vi "main.vi"() -> ()   [LabVIEW 2025]
uses:
  <userlib>/_NEVSTOP/Communicable State Machine(CSM)/Communicable State Machine.lvlib
  9e748aeb-3768-48be-8dba-7a0c5cfaea59.vi
  93a68443-ce49-4d48-b9a9-034adad3285b.vi
  780328b8-20a8-4e4e-91e5-c479b507fea7.vi
  <userlib>/_NEVSTOP/Communicable State Machine(CSM)/_Polymophic/Build Status Broadcast Message.vi
panel:
  out "Monitor":picture
  out "Error Occurred":errorcluster
  out "State History":string
  in  "Name (\"\" to Use UUID)":string="main"
  in  "Exit":bool
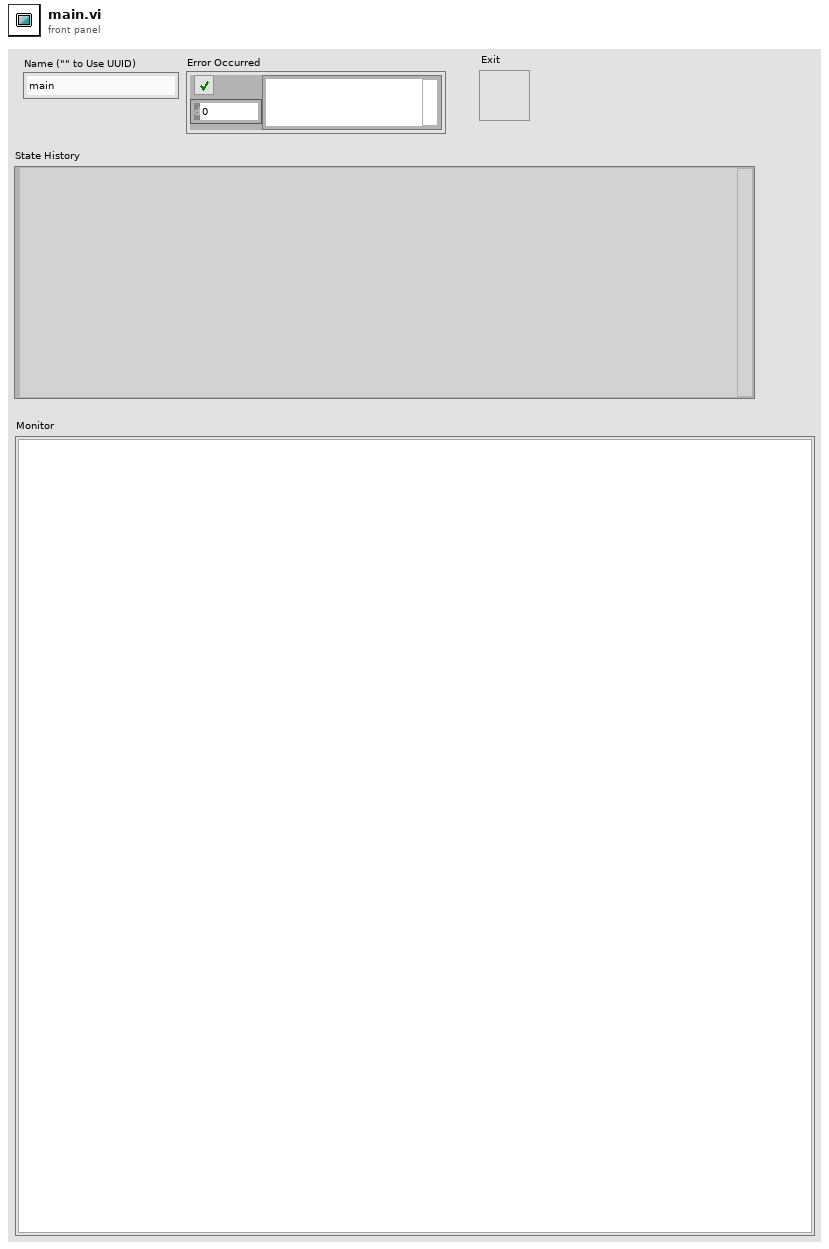
[diagram p1: front panel]
types:
  T1 = enum32{"Invalid", "Standard", "Closed", "Hidden", "Minimized", "Maximized"}
  T2 = enum32{"invalid app kind", "Development System", "Run Time System", "Student Edition", "Embedded LabVIEW", "Evaluation", "Custom"}
  T3 = cluster{"left":i16, "top":i16, "right":i16, "bottom":i16}
  T4 = typedef "Communicable State Machine.lvlib/_CSM_Response Source Message.ctl" = cluster{"‘State":string, "’Arguments":string, "’Error":errorcluster}
  T5 = typedef "eventvkey.ctl" = enum16{"ASCII", "Enter", "Return", "Shift", "Ctrl", "Alt", "Cmd", "Opt", "Caps", "NumLock", "Clear", "Break", "Up", "Down", "Left", "Right", "Insert", "Delete", "Home", "End", "PageUp", "PageDown", "Escape", "Help", "Pause", "ScrollLock", "F1", "F2", "F3", "F4", "F5", "F6", "F7", "F8", "F9", "F10", "F11", "F12", "F13", "F14", "F15", "F16", "F17", "F18", "F19", "F20", "F21", "F22", "F23", "F24", "Play", "VolumeUp", "VolumeDown", "Mute", "Two Byte Char"}
  T6 = cluster{"Current VI Reference":refnum<vi>, "Close Panel on Exit?":bool}
  T7 = cluster{"Core":cluster{"Current VI Reference":refnum<vi>, "Close Panel on Exit?":bool}, "player":cluster{"left":i16, "top":i16, "right":i16, "bottom":i16}, "Top Left Walll":cluster{"x":i16, "y":i16}[], "Top Right Walll":cluster{"x":i16, "y":i16}[], "Down Left Walll":cluster{"x":i16, "y":i16}[], "Down RightWalll":cluster{"x":i16, "y":i16}[], "Monitor":picture, "Gate Up":cluster{"left":i16, "top":i16, "right":i16, "bottom":i16}, "Gate Down":cluster{"left":i16, "top":i16, "right":i16, "bottom":i16}, "Gate Left":cluster{"left":i16, "top":i16, "right":i16, "bottom":i16}, "Gate Right":cluster{"left":i16, "top":i16, "right":i16, "bottom":i16}, "Gate Condition":bool[], "Level":i32}
  T8 = cluster{"left":i16, "top":i16, "right":i16, "bottom":i16}[]
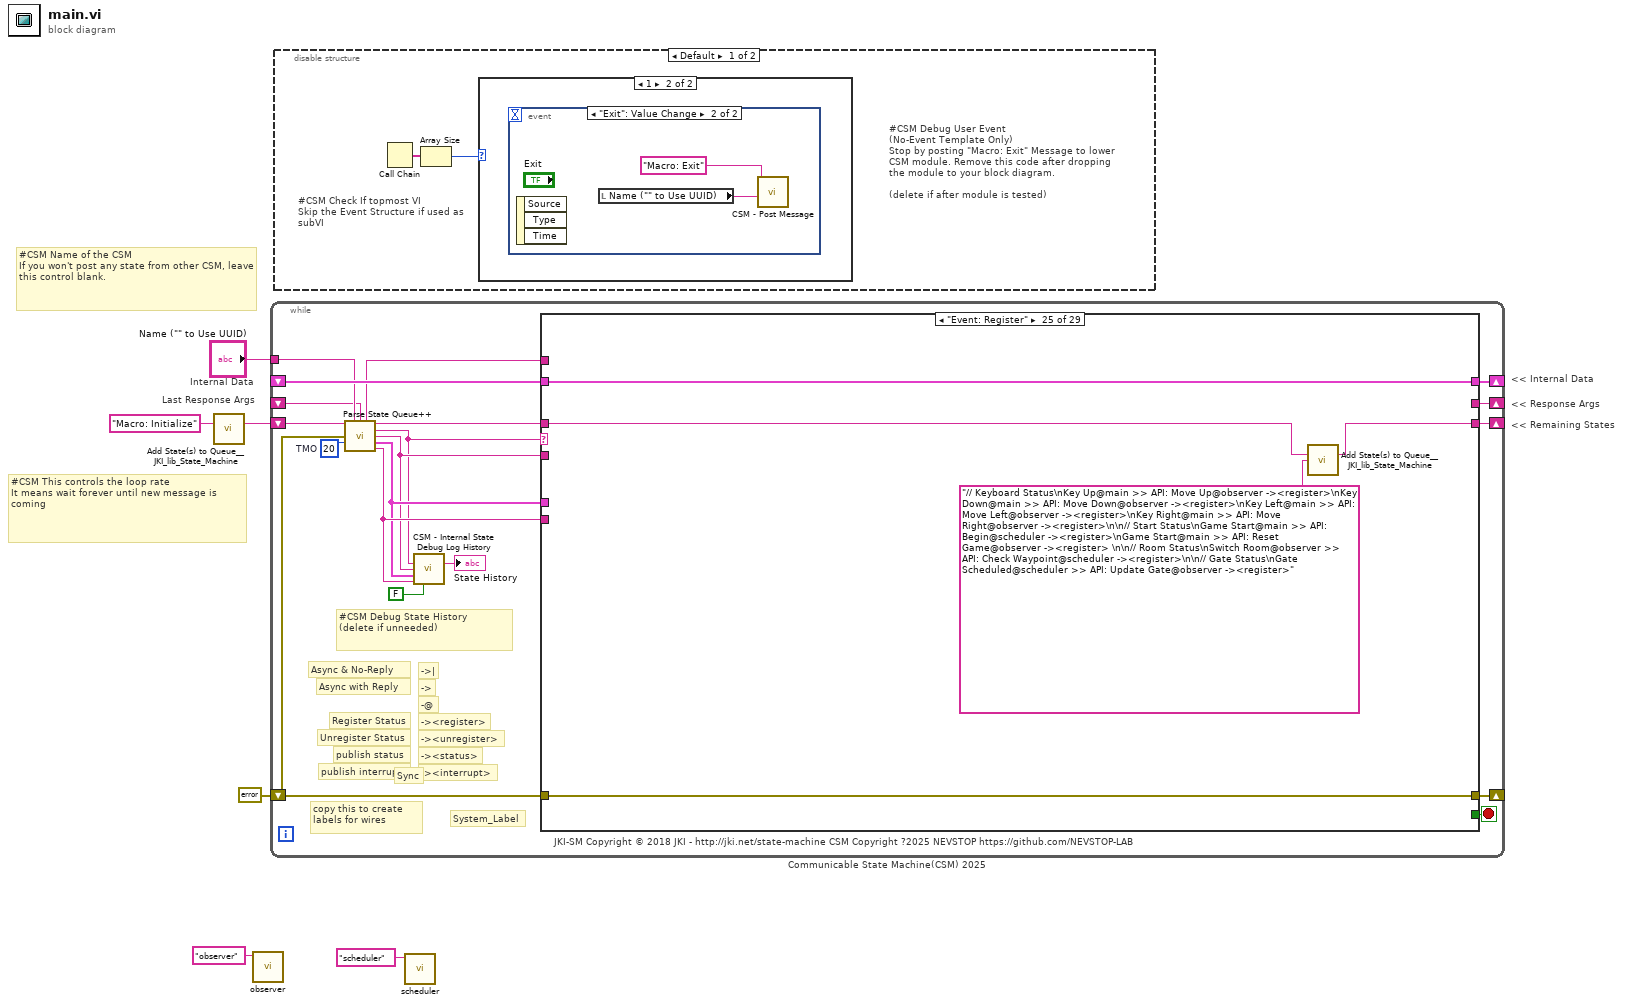
[diagram p0: block diagram]
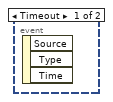
[diagram p3: hidden frame]
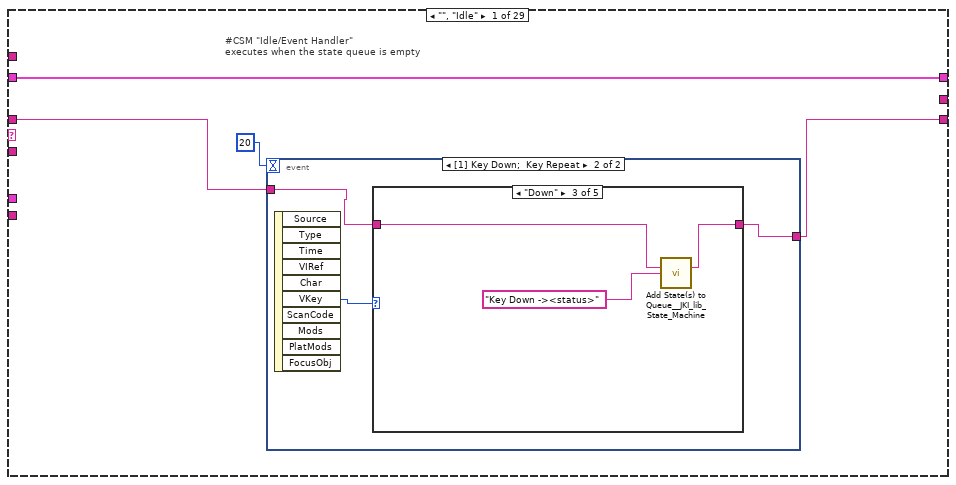
[diagram p5: hidden frame]
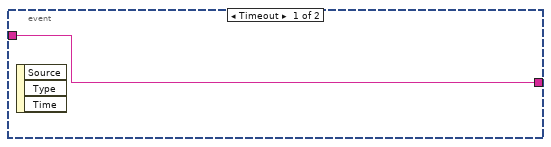
[diagram p6: hidden frame]
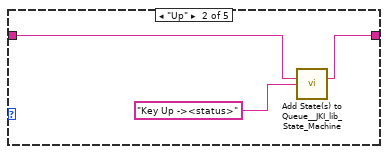
[diagram p8: hidden frame]
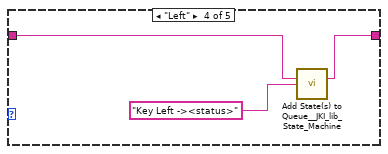
[diagram p9: hidden frame]
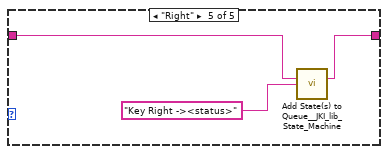
[diagram p10: hidden frame]
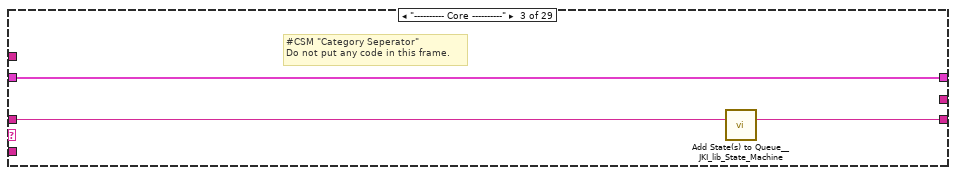
[diagram p12: hidden frame]
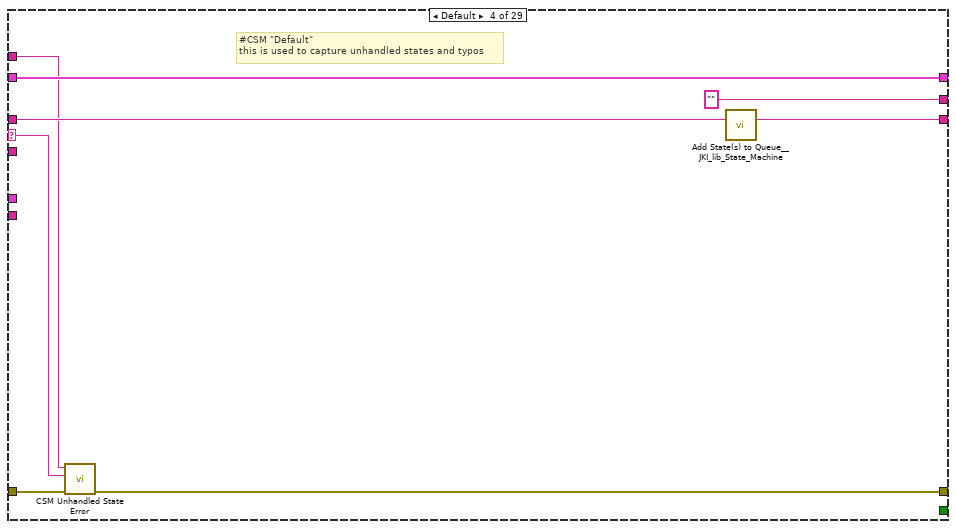
[diagram p13: hidden frame]
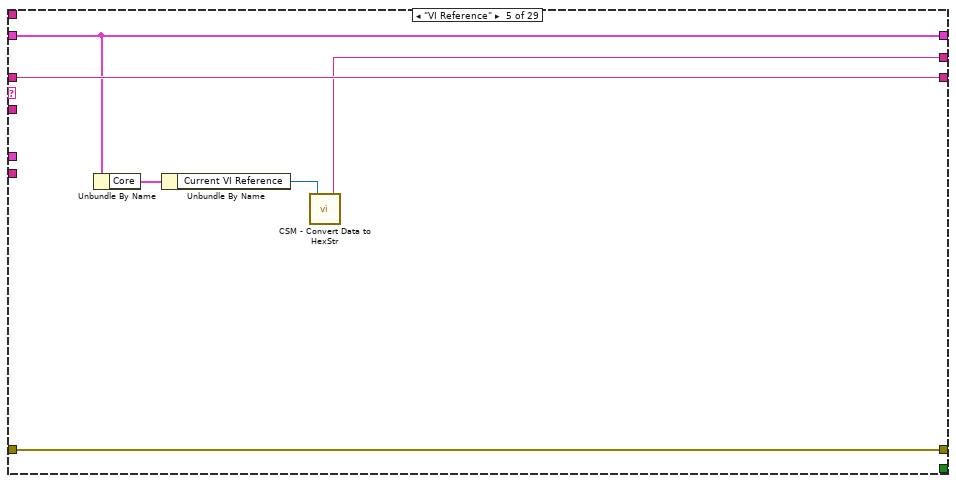
[diagram p14: hidden frame]
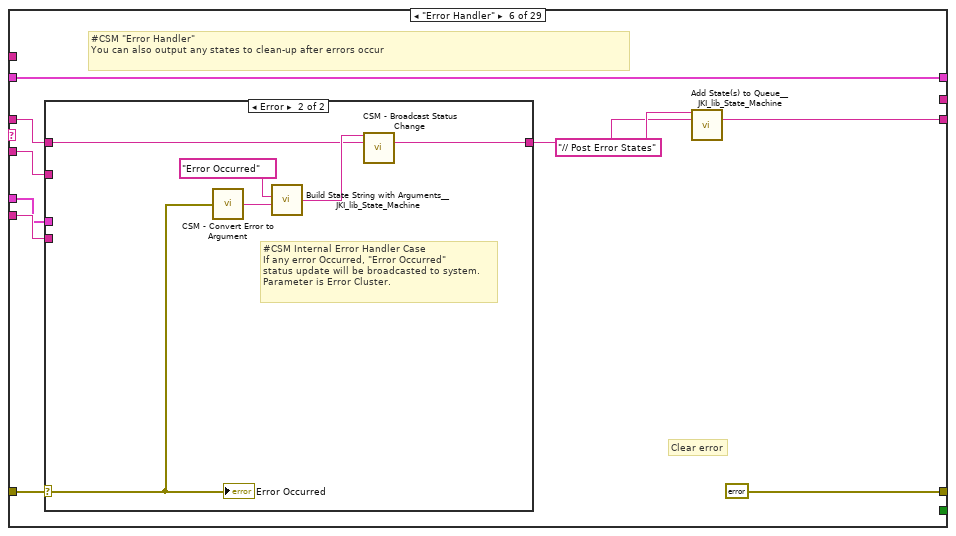
[diagram p15: hidden frame]
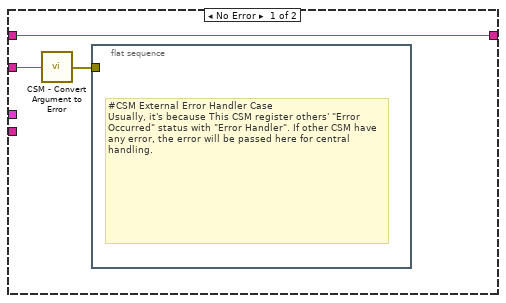
[diagram p16: hidden frame]
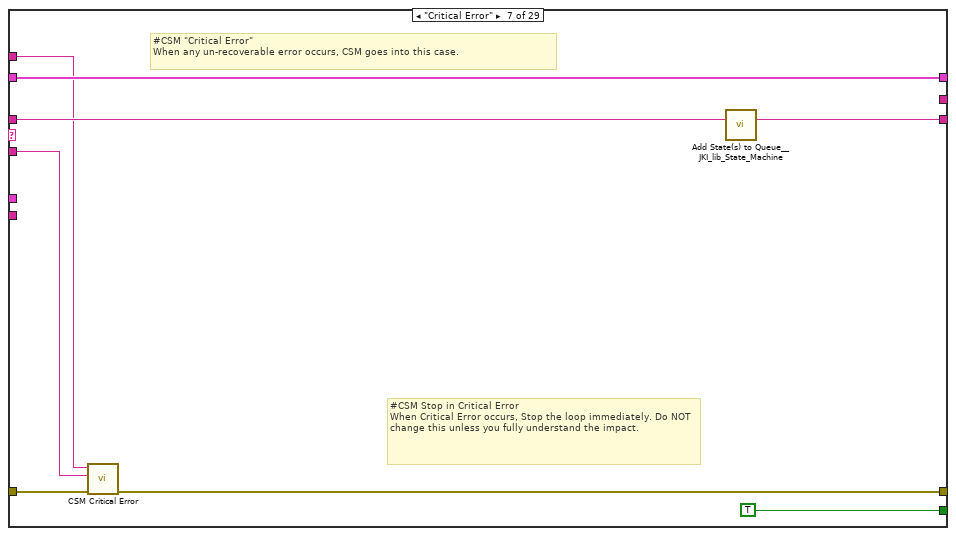
[diagram p17: hidden frame]
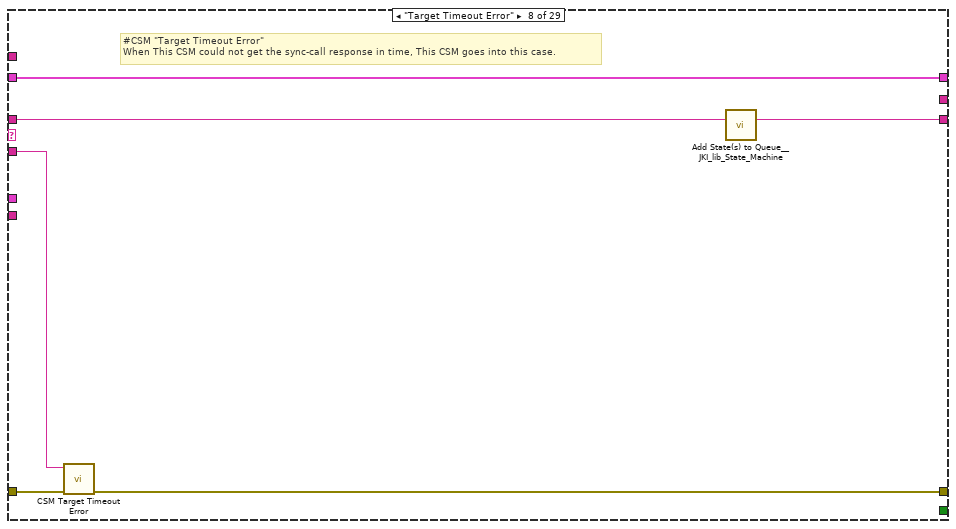
[diagram p18: hidden frame]
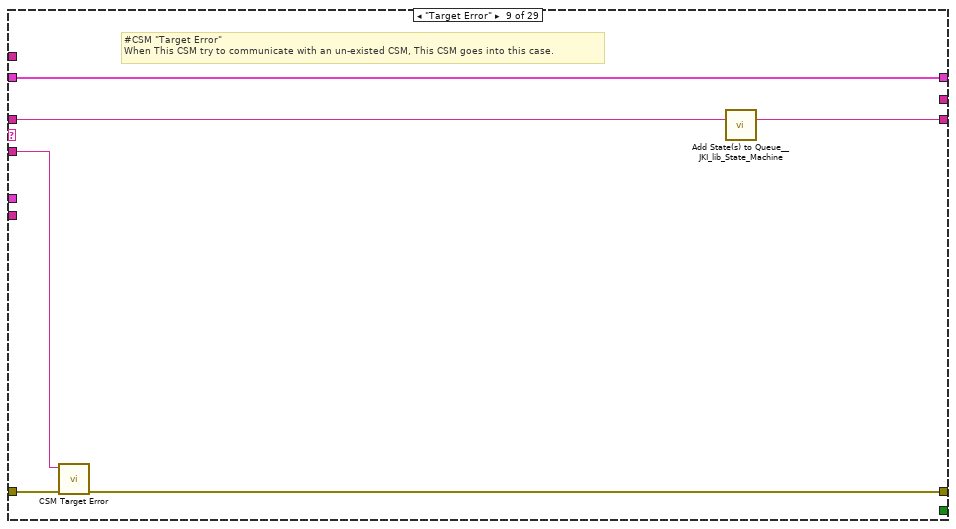
[diagram p19: hidden frame]
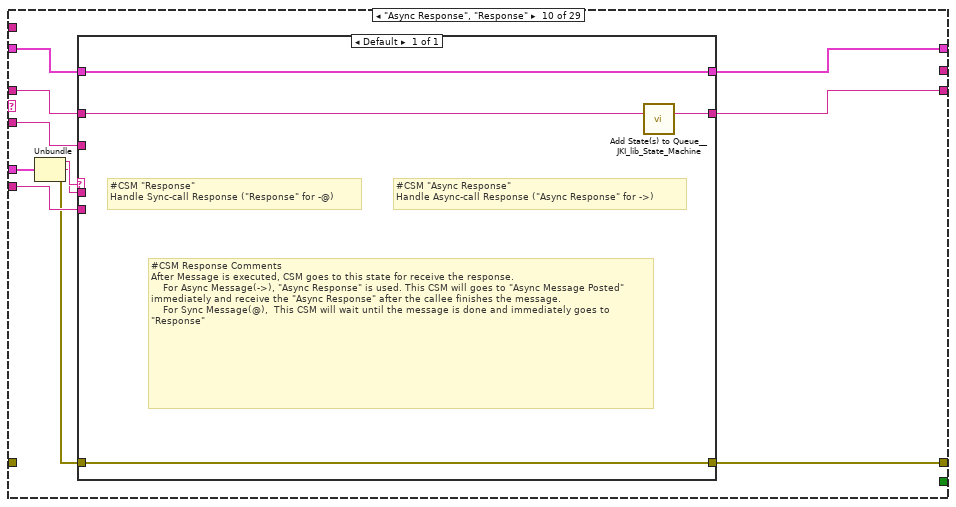
[diagram p20: hidden frame]
diagram:
  # "Last Response Args"
  # "Internal Data"
  # "#CSM Name of the CSM\nIf you won't post any state from other CSM, leave this control blank."
  # "#CSM This controls the loop rate\nIt means wait forever until new message is coming"
  # "<< Internal Data"
  # "<< Response Args"
  # "<< Remaining States"
  n1 = call <vilib>:"Add State(s) to Queue__JKI_lib_State_Machine.vi"("State(s) in (\"\")"="Macro: Initialize" ("Init State(\"Macro: Initialize\")")) -> ("States Out"=w3:string)  [unwired: 14 in]
  n2 = call "observer.vi"("Name (\"\" to Use UUID)"="observer" ("Name (\"\" to Use UUID)")) -> ()  [unwired: 11 in]
  n3 = while "Communicable State Machine(CSM) 2025" {
    shift-right: [w20] -> _
    shift-left: _ -> [w19]
    shift-right: [w23] -> _
    shift-left: errorcluster {"status"=FALSE, "code"=0, "source"=""} ("error out") -> [w9]
    shift-right: [w22] -> _
    shift-left: w3 -> [w24]
    tunnel: "Name (\"\" to Use UUID)" -> [w16]
    shift-right: [w17] -> _
    shift-left: _ -> [w11]
    stop <- w21 stop-if-true
    w18 = 20  # TMO
    # "#CSM Debug State History\n(delete if unneeded)"
    # "-><interrupt>"
    # "-><status>"
    # "-><unregister>"
    # "-><register>"
    # "-@"
    # "->"
    # "->|"
    # "publish interrupt"
    # "publish status"
    # "Unregister Status"
    # "Register Status"
    # "Sync"
    # "Async with Reply"
    # "Async & No-Reply"
    # "JKI-SM Copyright © 2018 JKI - http://jki.net/state-machine CSM Copyright ?2025 NEVSTOP https://github.com/NEVSTOP-LAB"
    # "copy this to create labels for wires"
    # "System_Label"
    n4 = call <userlib>:"Parse State Queue++.vi"("State Queue"=w24, "Name (\"\" to Use UUID)"=w16, "Response Arguments"=w11, "Previous Error"=w9, "Dequeue (1 ms)"=w18) -> ("Name Used"=w10:string, "Remaining States"=w25:string, "Current State"=w12:string, "Arguments"=w13:string, "Additional Information"=w14:T4, "Source CSM"=w15:string)  [unwired: 5 in]
    n5 = call <userlib>:"CSM - Internal State Debug Log History.vi"("State"=w12, "Arguments (\"\")"=w13, ">> Response Source Message >>"=w14, "Source (\"\")"=w15, "Enable Periodic State Filter? (T)"=FALSE) -> ("Debug Log"=→"State History":string)  [unwired: 10 in]
    n6 = case shown="\"Event: Register\"" w12 {
      selector: w12 -> [_ _ _ w55 _ _ _ _ _ _ _ _ _ _ _ _ _ _ _ _ _ _ _ _ _ _ _ _ _]
      tunnel: w25 -> [w27 w48 w51 w59 w64 w69 w92 w98 w104 w114 w121 w133 w137 w140 w156 w158 w164 w166 w168 w205 w209 w223 w230 w232 w236 w240 w243 w252 w261]
      tunnel: w13 -> [_ _ _ _ _ w68 w88 w95 w101 w108 _ _ _ _ _ _ _ _ _ _ _ _ _ _ _ _ _ w250 w259]
      tunnel: w19 -> [w29 w47 w49 w57 w63 w74 w90 w96 w102 w112 w120 w127 w135 w138 _ w157 w159 w165 w181 w203 w207 w222 w228 w231 w237 w239 w242 w247 w257]
      tunnel: [_ _ _ w52 w65 errorcluster {"status"=FALSE, "code"=0, "source"=""} ("error out") w85 w93 w99 w115 _ _ _ _ _ _ w160 w167 w188 _ _ w224 _ w233 w238 w241 _ _ _] -> w23
      tunnel: w9 -> [_ _ _ w53 w65 w72 w86 w94 w100 _ _ _ _ _ _ _ w161 w167 w188 _ _ w224 _ w233 w238 w241 _ _ _]
      tunnel: [w26 w48 w50 w58 w64 w70 w91 w97 w103 w113 w121 w132 w136 w139 w155 w158 w163 w166 w168 w204 w208 w211 w229 w232 w235 w240 w243 w251 w260] -> w22
      tunnel: [_ _ _ _ _ _ TRUE _ _ _ _ _ TRUE _ _ _ _ _ _ _ _ _ _ _ _ _ _ _ _] -> w21
      tunnel: [w29 w47 w49 w57 w63 w74 w90 w96 w102 w111 w120 w131 w135 w138 w154 w157 w159 w165 w180 w203 w207 w221 w228 w231 w237 w239 w242 w246 w256] -> w20
      tunnel: w15 -> [_ _ _ _ _ w67 _ _ _ w109 _ _ _ _ _ _ _ _ _ _ _ _ _ _ _ _ _ _ _]
      tunnel: w14 -> [_ _ _ _ _ w66 _ _ _ w110 _ _ _ _ _ _ _ _ _ _ _ _ _ _ _ _ _ _ _]
      tunnel: [_ _ _ "" w60 _ _ _ _ _ _ _ _ _ _ _ _ _ _ _ _ "Game Started" ("HEX String (0-9,A-F)") _ _ _ _ _ "Position Updated" ("HEX String (0-9,A-F)") "Gate Updated" ("HEX String (0-9,A-F)")] -> w17
      tunnel: w10 -> [_ _ _ w54 _ _ w87 _ _ _ _ _ _ _ _ _ _ _ _ _ _ _ _ _ _ _ _ _ _]
      frame "", "Idle" {
        # "#CSM \"Idle/Event Handler\"\nexecutes when the state queue is empty"
        n7 = event shown="[1] Key Down;  Key Repeat" {
          selector: _ -> [_ _]
          dyn-events: _ -> [_ _]
          timeout: 20 -> [_ _]
          tunnel: w27 -> [w30 w33]
          tunnel: [w30 w32] -> w26
          event Timeout {
            n8 = event-data() -> ()  [unwired: 1 in, 3 out]
          }
          event Key Down; Key Repeat {
            n9 = event-data() -> ("VKey"=w31:T5)  [unwired: 1 in, 9 out]
            n10 = case shown="\"Down\"" w31 {
              tunnel: w33 -> [w34 w37 w40 w43 w46]
              tunnel: [w34 w36 w39 w42 w45] -> w32
              frame "ASCII", Default {
              }
              frame "Up" {
                n11 = call <vilib>:"Add State(s) to Queue__JKI_lib_State_Machine.vi"("State(s) in (\"\")"=w37, "State(s) at Back (\"\")"="Key Up -><status>" ("State(s) at Back (\"\")")) -> ("States Out"=w36:string)  [unwired: 13 in]
              }
              frame "Down" {
                n12 = call <vilib>:"Add State(s) to Queue__JKI_lib_State_Machine.vi"("State(s) in (\"\")"=w40, "State(s) at Back (\"\")"="Key Down -><status>" ("State(s) at Back (\"\")")) -> ("States Out"=w39:string)  [unwired: 13 in]
              }
              frame "Left" {
                n13 = call <vilib>:"Add State(s) to Queue__JKI_lib_State_Machine.vi"("State(s) in (\"\")"=w43, "State(s) at Back (\"\")"="Key Left -><status>" ("State(s) at Back (\"\")")) -> ("States Out"=w42:string)  [unwired: 13 in]
              }
              frame "Right" {
                n14 = call <vilib>:"Add State(s) to Queue__JKI_lib_State_Machine.vi"("State(s) in (\"\")"=w46, "State(s) at Back (\"\")"="Key Right -><status>" ("State(s) at Back (\"\")")) -> ("States Out"=w45:string)  [unwired: 13 in]
              }
            }
          }
        }
      }
      frame "CSM Documentation" {
        # "#CSM State Syntax\n\n// Comment line, all text to the right of “//” will be ignored\n// Local Message Example\nDoSth: DoA >> Arguments\n\n// Sync Call Example\nAPI: xxxx >> Arguments -@ TargetModule\n\n// Async Call Example\nAPI: xxxx >> Arguments -> TargetModule\n\n// Async Call without Reply Example\nAPI: xxxx >> Arguments ->| TargetModule\n\n// Broadcast normal status:\nStatus >> StatusArguments  -><status>\n\n// Broadcast Interrupt status:\nInterrupt >> StatusArguments  -><interrupt>\n\n// Register Source Module's status to Handler Module\nStatus@Source Module >> Handler Module@Handler Module -><register>\n\n// Unegister Source Module's status\nStatus@Source Module >> Handler Module -><unregister>"
        # "#CSM README FIRST\n\nCommunicable State Machine(CSM) is a LabVIEW application framework that builds upon JKI State Machine(JKISM). It follows the pattern of JKISM and extends the keywords to describe message communication between modules, including concepts such as Sync-Message, Async-Message, Subscription/Unsubscription of status - essential elements for creating reusable code modules. For more information, please visit the CSM wiki: https://nevstop-lab.github.io/CSM-Wiki/\n\nFor instructions on JKI State Machine, visit: \n    http://jki.net/state-machine/\nFor information about CSM, visit: \n    https://github.com/NEVSTOP-LAB"
        # "#CSM \"Documentation\"\nCase for holding CSM Documenation"
      }
      frame "---------- Core ----------" {
        # "#CSM \"Category Seperator\"\nDo not put any code in this frame."
        n15 = call <vilib>:"Add State(s) to Queue__JKI_lib_State_Machine.vi"("State(s) in (\"\")"=w51) -> ("States Out"=w50:string)  [unwired: 14 in]
      }
      frame Default {
        # "#CSM \"Default\"\nthis is used to capture unhandled states and typos"
        n16 = call <userlib>:"CSM Unhandled State Error.vi"("error in (no error)"=w53, "Undefined State"=w55, "CSM Name"=w54) -> ("error out"=w52:errorcluster)  [unwired: 8 in]
        n17 = call <vilib>:"Add State(s) to Queue__JKI_lib_State_Machine.vi"("State(s) in (\"\")"=w59) -> ("States Out"=w58:string)  [unwired: 14 in]
      }
      frame "VI Reference" {
        n18 = Unbundle By Name(w63) -> ("Core"=w62:T6)
        n19 = Unbundle By Name(w62) -> ("Current VI Reference"=w61:refnum<vi>)
        n20 = call <userlib>:"CSM - Convert Data to HexStr.vi"("Variant"=w61) -> ("HEX String (0-9,A-F)"=w60:string)  [unwired: 8 in]
      }
      frame "Error Handler" {
        # "#CSM \"Error Handler\"\nYou can also output any states to clean-up after errors occur"
        # "Clear error"
        n21 = case shown="Error" w72 {
          selector: w72 -> [_ w79]
          tunnel: [w78 w81] -> w71
          tunnel: w69 -> [w78 w80]
          tunnel: w68 -> [w77 _]
          tunnel: w67 -> [_ _]
          tunnel: w66 -> [_ _]
          frame No Error {
            n22 = call <userlib>:"CSM - Convert Argument to Error.vi"("Argument"=w77) -> ("Error"=w76:errorcluster)  [unwired: 4 in]
            n23 = flat-sequence {
              tunnel: w76 -> [_]
              frame #0 {
                # "#CSM External Error Handler Case\nUsually, it's because This CSM register others' \"Error Occurred\" status with \"Error Handler\". If other CSM have any error, the error will be passed here for central handling."
              }
            }
          }
          frame Error {
            # "#CSM Internal Error Handler Case \nIf any error Occurred, \"Error Occurred\" \nstatus update will be broadcasted to system.\nParameter is Error Cluster."
            n24 = call <userlib>:"CSM - Convert Error to Argument.vi"("Error"=w79) -> ("Argument"=w83:string)  [unwired: 4 in]
            n25 = call <vilib>:"Build State String with Arguments__JKI_lib_State_Machine.vi"("Arguments (\"\")"=w83, "State"="Error Occurred" ("Status with Arguments")) -> ("State with Arguments"=w82:string)  [unwired: 4 in]
            n26 = call <userlib>:"CSM - Broadcast Status Change.vi"("Status With Arguments"=w82, "State Queue"=w80) -> ("Remaining States"=w81:string)  [unwired: 13 in]
            "Error Occurred" <- w79
          }
        }
        n27 = call <vilib>:"Add State(s) to Queue__JKI_lib_State_Machine.vi"("State(s) in Front (\"\")"="// Post Error States", "State(s) in (\"\")"=w71) -> ("States Out"=w70:string)  [unwired: 13 in]
      }
      frame "Critical Error" {
        # "#CSM \"Critical Error\"\nWhen any un-recoverable error occurs, CSM goes into this case."
        # "#CSM Stop in Critical Error\nWhen Critical Error occurs, Stop the loop immediately. Do NOT change this unless you fully understand the impact."
        n28 = call <userlib>:"CSM Critical Error.vi"("error in (no error)"=w86, "Arugments (As Reason)"=w88, "CSM Name"=w87) -> ("error out"=w85:errorcluster)  [unwired: 8 in]
        n29 = call <vilib>:"Add State(s) to Queue__JKI_lib_State_Machine.vi"("State(s) in (\"\")"=w92) -> ("States Out"=w91:string)  [unwired: 14 in]
      }
      frame "Target Timeout Error" {
        # "#CSM \"Target Timeout Error\"\nWhen This CSM could not get the sync-call response in time, This CSM goes into this case."
        n30 = call <userlib>:"CSM Target Timeout Error.vi"("error in (no error)"=w94, "Arguments (As CSM Name)"=w95) -> ("error out"=w93:errorcluster)  [unwired: 9 in]
        n31 = call <vilib>:"Add State(s) to Queue__JKI_lib_State_Machine.vi"("State(s) in (\"\")"=w98) -> ("States Out"=w97:string)  [unwired: 14 in]
      }
      frame "Target Error" {
        # "#CSM \"Target Error\"\nWhen This CSM try to communicate with an un-existed CSM, This CSM goes into this case."
        n32 = call <userlib>:"CSM Target Error.vi"("error in (no error)"=w100, "Arguments (As CSM Name)"=w101) -> ("error out"=w99:errorcluster)  [unwired: 9 in]
        n33 = call <vilib>:"Add State(s) to Queue__JKI_lib_State_Machine.vi"("State(s) in (\"\")"=w104) -> ("States Out"=w103:string)  [unwired: 14 in]
      }
      frame "Async Response", "Response" {
        n34 = Unbundle(w110) -> ("‘State"=w107:string, "’Arguments"=w106:string, "’Error"=w105:errorcluster)
        n35 = case shown="Default" w107 {
          tunnel: [w116] -> w113
          tunnel: w114 -> [w117]
          tunnel: [w119] -> w111
          tunnel: w112 -> [w119]
          tunnel: [w118] -> w115
          tunnel: w105 -> [w118]
          tunnel: w109 -> [_]
          tunnel: w108 -> [_]
          tunnel: w106 -> [_]
          frame Default {
            # "#CSM \"Async Response\"\nHandle Async-call Response (\"Async Response\" for ->)"
            # "#CSM \"Response\"\nHandle Sync-call Response (\"Response\" for -@)"
            # "#CSM Response Comments\nAfter Message is executed, CSM goes to this state for receive the response.\n    For Async Message(->), \"Async Response\" is used. This CSM will goes to \"Async Message Posted\" immediately and receive the \"Async Response\" after the callee finishes the message.\n    For Sync Message(@),  This CSM will wait until the message is done and immediately goes to \"Response\""
            n36 = call <vilib>:"Add State(s) to Queue__JKI_lib_State_Machine.vi"("State(s) in (\"\")"=w117) -> ("States Out"=w116:string)  [unwired: 14 in]
          }
        }
      }
      frame "Async Message Posted" {
        # "#CSM \"Async Message Posted\"\nAfter Async Message is posted (-> or ->| ), CSM goes to this state for post-action.\nYou can use Argument - State to tell which Async Message is called."
      }
      frame "Initialize Core Data" {
        # "#CSM \"Initialize Core Data\"\nThis is used to determine panel behavior on exit"
        # "originally closed?"
        # "exe?"
        # "If panel starts closed or is an EXE, then close it when we exit"
        n37 = control-ref of="Current VI Reference"() -> (w125:refnum<vi>)
        n38 = property class="VI"() -> ("FP.State"=w124:T1)  [unwired: 2 in, 2 out]
        n39 = property class="App"() -> ("App.Kind"=w130:T2)  [unwired: 2 in, 2 out]
        n40 = Equal?(x=w124, y=T1."Closed" ("Front Panel Window:State")) -> (x = y?=w122:bool)
        n41 = Equal?(x=w130, y=T2."Run Time System" ("Application:Kind")) -> (x = y?=w128:bool)
        n42 = Or(x=w122, y=w128) -> (x .or. y?=w126:bool)
        n43 = Bundle By Name(cluster=w127, "Core.Current VI Reference"=w125, "Core.Close Panel on Exit?"=w126) -> (w131:T7)
        n44 = call <vilib>:"Add State(s) to Queue__JKI_lib_State_Machine.vi"("State(s) in (\"\")"=w133) -> ("States Out"=w132:string)  [unwired: 14 in]
      }
      frame "Exit" {
        # "#CSM \"Exit\"\nCase for exiting the loop. No errors that occur here will be handled."
        n45 = call <vilib>:"Add State(s) to Queue__JKI_lib_State_Machine.vi"("State(s) in (\"\")"=w137) -> ("States Out"=w136:string)  [unwired: 14 in]
      }
      frame "---------- Data ----------" {
        # "#CSM \"Category Seperator\"\nDo not put any code in this frame."
        n46 = call <vilib>:"Add State(s) to Queue__JKI_lib_State_Machine.vi"("State(s) in (\"\")"=w140) -> ("States Out"=w139:string)  [unwired: 14 in]
      }
      frame "Data: Initialize" {
        w141 = 0  # Level
        w142 = bool[] [FALSE, FALSE, FALSE, FALSE]  # Gate Condition
        w143 = T3 {"left"=750, "top"=325, "right"=800, "bottom"=475}  # Gate Right
        w144 = T3 {"left"=0, "top"=325, "right"=50, "bottom"=475}  # Gate Left
        w145 = T3 {"left"=325, "top"=750, "right"=475, "bottom"=800}  # Gate Down
        w146 = T3 {"left"=325, "top"=0, "right"=475, "bottom"=50}  # Gate Up
        w147 = picture data[5B]  # Monitor
        w148 = T3 {"left"=375, "top"=375, "right"=425, "bottom"=425}  # player
        w149 = cluster{"x":i16, "y":i16}[] [{"x"=475, "y"=750}, {"x"=750, "y"=750}, {"x"=750, "y"=475}, {"x"=800, "y"=475}, {"x"=800, "y"=800}, {"x"=475, "y"=800}]  # Down RightWalll
        w150 = cluster{"x":i16, "y":i16}[] [{"x"=0, "y"=475}, {"x"=50, "y"=475}, {"x"=50, "y"=750}, {"x"=325, "y"=750}, {"x"=325, "y"=800}, {"x"=0, "y"=800}]  # Down Left Walll
        w151 = cluster{"x":i16, "y":i16}[] [{"x"=475, "y"=0}, {"x"=800, "y"=0}, {"x"=800, "y"=325}, {"x"=750, "y"=325}, {"x"=750, "y"=50}, {"x"=475, "y"=50}]  # Top Right Walll
        w152 = cluster{"x":i16, "y":i16}[] [{"x"=0, "y"=0}, {"x"=325, "y"=0}, {"x"=325, "y"=50}, {"x"=50, "y"=50}, {"x"=50, "y"=325}, {"x"=0, "y"=325}]  # Top Left Walll
        w153 = T6 {"Current VI Reference"=refnum, "Close Panel on Exit?"=FALSE}  # Core
        # "#CSM \"Data: Initialize\"\nInitialize the shift-register data, here.\n(data names are defined by what you wire into the bundle function)"
        # "#CSM do not delete - used by framework"
        n47 = call <vilib>:"Add State(s) to Queue__JKI_lib_State_Machine.vi"("State(s) in (\"\")"=w156) -> ("States Out"=w155:string)  [unwired: 14 in]
        n48 = Bundle("Core"=w153, "player"=w148, "Top Left Walll"=w152, "Top Right Walll"=w151, "Down Left Walll"=w150, "Down RightWalll"=w149, "Monitor"=w147, "Gate Up"=w146, "Gate Down"=w145, "Gate Left"=w144, "Gate Right"=w143, "Gate Condition"=w142, "Level"=w141) -> (w154:T7)  [unwired: 1 in]
      }
      frame "Data: Update Indicators" {
      }
      frame "Data: Cleanup" {
        # "#CSM \"Data: Cleanup\"\nCleanup any data and references, here.\n(this is called automatically, by the Macro: Exit)"
        n49 = Unbundle By Name(w159) -> ("Core.Current VI Reference"=w162:refnum<vi>)
        n50 = Close Reference(reference=w162, error in (no error)=w161) -> (error out=w160:errorcluster)
        n51 = call <vilib>:"Add State(s) to Queue__JKI_lib_State_Machine.vi"("State(s) in (\"\")"=w164) -> ("States Out"=w163:string)  [unwired: 14 in]
      }
      frame "---------- UI ----------" {
      }
      frame "UI: Update" {
        w169 = picture data[5B]  # Monitor
        w176 = TRUE ("fill?(F)")
        n52 = Unbundle By Name(w181) -> ("Top Left Walll"=w187:cluster{"x":i16, "y":i16}[], "Top Right Walll"=w186:cluster{"x":i16, "y":i16}[], "Down Left Walll"=w185:cluster{"x":i16, "y":i16}[], "Down RightWalll"=w184:cluster{"x":i16, "y":i16}[], "player"=w182:T3, "Gate Condition"=w170:bool[], "Gate Up"=w175:T3, "Gate Down"=w174:T3, "Gate Left"=w173:T3, "Gate Right"=w172:T3)
        n53 = Build Array(w175, w174, w173, w172) -> (w171:T8)
        n54 = Build Array(w187, w186, w185, w184) -> (w183:cluster{"x":i16, "y":i16}[][])
        n55 = for {
          tunnel: w183 -> [w201] mode=indexing
          tunnel: w176 -> [w200]
          shift-right: [w199] -> w178
          shift-left: w169 -> [w202]
          n56 = call <vilib>:"Draw Multiple Lines.vi"("picture"=w202, "line endpoints"=w201, "fill?(F)"=w200) -> ("new picture"=w199:picture)  [unwired: 6 in]
        }
        n57 = for {
          shift-right: [w192] -> w177
          shift-left: w178 -> [w193]
          tunnel: w176 -> [w191]
          tunnel: w171 -> [w190] mode=indexing
          tunnel: w170 -> [w189] mode=indexing
          n58 = case shown="True" w189 {
            tunnel: [w194 w195] -> w192
            tunnel: w193 -> [w194 w196]
            tunnel: w191 -> [_ w198]
            tunnel: w190 -> [_ w197]
            frame False {
            }
            frame True {
              n59 = call <vilib>:"Draw Rectangle.vi"("picture"=w196, "rect"=w197, "fill?(F)"=w198) -> ("new picture"=w195:picture)  [unwired: 6 in]
            }
          }
        }
        n60 = call <vilib>:"Draw Rectangle.vi"("picture"=w177, "rect"=w182, "fill?(F)"=w176) -> ("new picture"=w179:picture)  [unwired: 6 in]
        "Monitor" <- w179
        n61 = Bundle By Name(cluster=w181, "Monitor"=w179) -> (w180:T7)
      }
      frame "---------- Macro ----------" {
        # "#CSM \"Category Seperator\"\nDo not put any code in this frame."
        n62 = call <vilib>:"Add State(s) to Queue__JKI_lib_State_Machine.vi"("State(s) in (\"\")"=w205) -> ("States Out"=w204:string)  [unwired: 14 in]
      }
      frame "Macro: Initialize" {
        # "#CSM \"Macro: Initialize\"\nInitialization Macro (This is called once, when the VI starts)"
        n63 = call <vilib>:"Add State(s) to Queue__JKI_lib_State_Machine.vi"("State(s) in Front (\"\")"="Initialize Core Data\nData: Initialize\nEvent: Register\nMacro: Game Start\nData: Update Indicators", "State(s) in (\"\")"=w209) -> ("States Out"=w208:string)  [unwired: 13 in]
      }
      frame "Macro: Game Start" {
        w218 = bool[] [FALSE, FALSE, FALSE, FALSE]  # Gate Condition
        w219 = T3 {"left"=375, "top"=375, "right"=425, "bottom"=425}  # player
        n64 = Unbundle By Name(w222) -> ("Level"=w220:i32)
        n65 = Increment(x=w220) -> (x+1=w216:i32)
        n66 = Bundle By Name(cluster=w222, "Level"=w216, "player"=w219, "Gate Condition"=w218) -> (w221:T7)
        n67 = call "CSM - Convert MassData to Argument.vim"("Data"=w216) -> ("MassData Argument"=w215:string)  [unwired: 7 in, 1 out]
        n68 = call <vilib>:"Add State(s) to Queue__JKI_lib_State_Machine.vi"("State(s) in (\"\")"=w223, "State(s) at Back (\"\")"="UI: Update") -> ("States Out"=w213:string)  [unwired: 13 in]
        n69 = call-poly <userlib>:"Build Message with Arguments++.vi"("State With Arguments"="Game Start", "Arguments (\"\")"=w215) -> ("CSM Message String"=w212:string)  [unwired: 13 in]
        n70 = call <vilib>:"Add State(s) to Queue__JKI_lib_State_Machine.vi"("State(s) in (\"\")"=w213, "State(s) at Back (\"\")"=w212) -> ("States Out"=w211:string)  [unwired: 13 in]
      }
      frame "Macro: Exit" {
        # "#CSM \"Macro: Exit\"\nExit Macro (This is called once, when the VI exits)"
        n71 = call <vilib>:"Add State(s) to Queue__JKI_lib_State_Machine.vi"("State(s) in Front (\"\")"="Macro: Exit -@ observer\nMacro: Exit -@ scheduler", "State(s) at Back (\"\")"="\nData: Cleanup\nExit") -> ("States Out"=w226:string)  [unwired: 13 in]
        n72 = call <vilib>:"Add State(s) to Queue__JKI_lib_State_Machine.vi"("State(s) in Front (\"\")"=w226, "State(s) in (\"\")"=w230) -> ("States Out"=w229:string)  [unwired: 13 in]
      }
      frame "---------- Event ----------" {
      }
      frame "Event: Register" {
        n73 = call <vilib>:"Add State(s) to Queue__JKI_lib_State_Machine.vi"("State(s) in (\"\")"=w236, "State(s) at Back (\"\")"="// Keyboard Status\nKey Up@main >> API: Move Up@observer -><register>\nKey Down@main >> API: Move Down@observer -><register>\nKey Left@main >> API: Move Left@observer -><register>\nKey Right@main >> API: Move Right@observer -><register>\n\n// Start Status\nGame Start@main >> API: Begin@scheduler -><register>\nGame Start@main >> API: Reset Game@observer -><register> \n\n// Room Status\nSwitch Room@observer >> API: Check Waypoint@scheduler -><register>\n\n// Gate Status\nGate Scheduled@scheduler >> API: Update Gate@observer -><register>") -> ("States Out"=w235:string)  [unwired: 13 in]
      }
      frame "Event: Unregister" {
      }
      frame "---------- API ----------" {
        # "#CSM \"Category Seperator\"\nDo not put any code in this frame."
      }
      frame "API: Update Position" {
        # "#CSM API Example\nCopy/Rename this case for your own API"
        n74 = call "CSM - Convert Argument to MassData.vim"("Type"=T3 {"left"=0, "top"=0, "right"=0, "bottom"=0} ("rect"), "MassData Argument"=w250) -> ("Data"=w248:T3)  [unwired: 6 in, 1 out]
        n75 = Bundle By Name(cluster=w247, "player"=w248) -> (w246:T7)
        n76 = call <vilib>:"Add State(s) to Queue__JKI_lib_State_Machine.vi"("State(s) in (\"\")"=w252, "State(s) at Back (\"\")"="UI: Update" ("State(s) at Back (\"\")")) -> ("States Out"=w251:string)  [unwired: 13 in]
      }
      frame "API: Update Gate" {
        w253 = bool[] []  # Gate Condition
        # "#CSM API Example\nCopy/Rename this case for your own API"
        n77 = call "CSM - Convert Argument to MassData.vim"("Type"=w253, "MassData Argument"=w259) -> ("Data"=w258:bool[])  [unwired: 6 in, 1 out]
        n78 = Bundle By Name(cluster=w257, "Gate Condition"=w258) -> (w256:T7)
        n79 = call <vilib>:"Add State(s) to Queue__JKI_lib_State_Machine.vi"("State(s) in (\"\")"=w261, "State(s) at Back (\"\")"="UI: Update" ("State(s) at Back (\"\")")) -> ("States Out"=w260:string)  [unwired: 13 in]
      }
    }
  }
  n80 = disable-structure shown="Default" {
    frame condition #0 (active) {
      # "#CSM Check If topmost VI\nSkip the Event Structure if used as subVI"
      # "#CSM Debug User Event\n(No-Event Template Only)\nStop by posting \"Macro: Exit\" Message to lower CSM module. Remove this code after dropping the module to your block diagram. \n\n(delete if after module is tested)"
      n81 = Call Chain() -> (call chain=w263:string[])
      n82 = Array Size(array=w263) -> (size(s)=w262:i32)
      n83 = case shown="1" w262 {
        frame Default {
        }
        frame 1 {
          n84 = event shown="[1] \"Exit\": Value Change" {
            selector: _ -> [_ _]
            dyn-events: _ -> [_ _]
            timeout: _ -> [_ _]
            event Timeout {
              n85 = event-data() -> ()  [unwired: 1 in, 3 out]
            }
            event "Exit": Value Change {
              n86 = event-data() -> ()  [unwired: 1 in, 3 out]
              n87 = local read "Name (\"\" to Use UUID)"() -> (w265:string)
              n88 = call <userlib>:"CSM - Post Message.vi"("Target Module"=w265, "State"="Macro: Exit" ("States")) -> ()  [unwired: 9 in, 1 out]
            }
          }
        }
      }
    }
    frame condition #1 {
    }
  }
  n89 = call "scheduler.vi"("Name (\"\" to Use UUID)"="scheduler" ("Name (\"\" to Use UUID)")) -> ()  [unwired: 11 in]
